vi "Test_Get Meta Data.vi"() -> ()   [LabVIEW 2020, in "Measurement_lv_client.lvlib" / "Measurement_lv_client.lvclass"]
uses:
  Measurement_lv_client.lvclass
  RPC Messages/Measurement_v1_GetMetadataResponse/Measurement_v1_GetMetadataResponse_Data.ctl
  RPC Messages/Measurement_v1_MeasurementDetails/Measurement_v1_MeasurementDetails_Data.ctl
  RPC Messages/Measurement_v1_MeasurementParameters/Measurement_v1_MeasurementParameters_Data.ctl
  RPC Messages/Measurement_v1_ConfigurationParameter/Measurement_v1_ConfigurationParameter_Data.ctl
  RPC Messages/Measurement_v1_OutputParameter/Measurement_v1_OutputParameter_Data.ctl
  RPC Messages/Measurement_v1_UserInterfaceDetails/Measurement_v1_UserInterfaceDetails_Data.ctl
panel:
  out "Response Data":T1
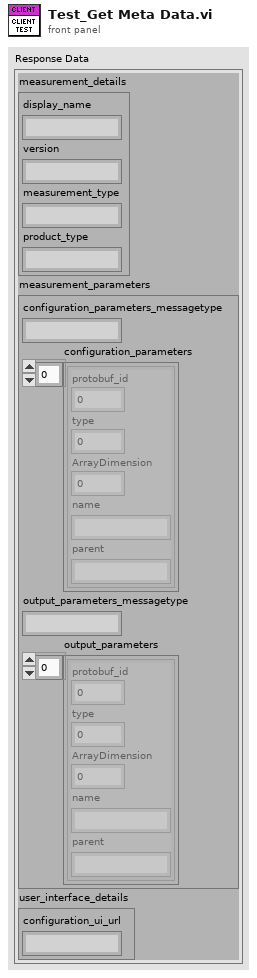
[diagram p1: front panel]
types:
  T1 = typedef "Measurement_lv_client.lvlib/Measurement_lv_client.lvclass/Measurement_v1_GetMetadataResponse_Data.ctl" = cluster{"measurement_details":T2, "measurement_parameters":T3, "user_interface_details":T6}
  T2 = typedef "Measurement_lv_client.lvlib/Measurement_lv_client.lvclass/Measurement_v1_MeasurementDetails_Data.ctl" = cluster{"display_name":string, "version":string, "measurement_type":string, "product_type":string}
  T3 = typedef "Measurement_lv_client.lvlib/Measurement_lv_client.lvclass/Measurement_v1_MeasurementParameters_Data.ctl" = cluster{"configuration_parameters_messagetype":string, "configuration_parameters":T4[], "output_parameters_messagetype":string, "output_parameters":T5[]}
  T4 = typedef "Measurement_lv_client.lvlib/Measurement_lv_client.lvclass/Measurement_v1_ConfigurationParameter_Data.ctl" = cluster{"protobuf_id":i32, "type":i32, "ArrayDimension":i32, "name":string, "parent":string}
  T5 = typedef "Measurement_lv_client.lvlib/Measurement_lv_client.lvclass/Measurement_v1_OutputParameter_Data.ctl" = cluster{"protobuf_id":i32, "type":i32, "ArrayDimension":i32, "name":string, "parent":string}
  T6 = typedef "Measurement_lv_client.lvlib/Measurement_lv_client.lvclass/Measurement_v1_UserInterfaceDetails_Data.ctl" = cluster{"configuration_ui_url":string}
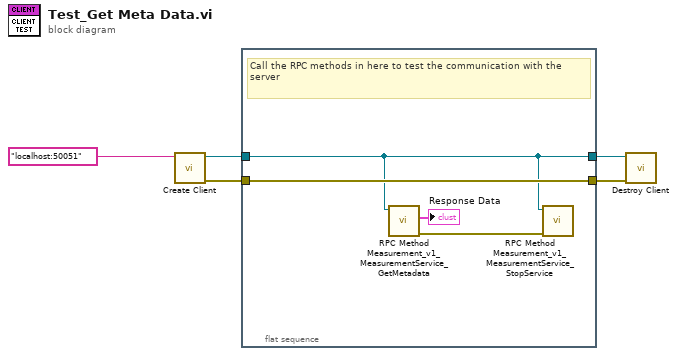
[diagram p0: block diagram]
diagram:
  n1 = call "Create Client.vi"("address"="localhost:50051") -> ("error out"=w1:errorcluster, "gRPC Client out"=w3:refnum<class "Measurement_lv_client.lvclass">)  [unwired: 9 in]
  n2 = flat-sequence {
    tunnel: [w6] -> w4
    tunnel: w3 -> [w6]
    tunnel: [w9] -> w2
    tunnel: w1 -> [w9]
    frame #0 {
      # "Call the RPC methods in here to test the communication with the server"
      n3 = call "RPC Method Measurement_v1_MeasurementService_GetMetadata.vi"("gRPC Client in"=w6) -> ("error out"=w7:errorcluster, "Response Data"=→"Response Data":T1)  [unwired: 8 in, 1 out]
      n4 = call "RPC Method Measurement_v1_MeasurementService_StopService.vi"("error in (no error)"=w7, "gRPC Client in"=w6) -> ()  [unwired: 7 in, 3 out]
    }
  }
  n5 = call "Destroy Client.vi"("error in (no error)"=w2, "gRPC Client in"=w4) -> ()  [unwired: 8 in, 2 out]
